vi "ROS_Wait.vi"(3 "milliseconds to wait":u32, 6 "error in":errorcluster) -> (5 "error out":errorcluster)   [LabVIEW 2010]
doc: "ROS for LV formatted wrapper for Wait(ms).vi"
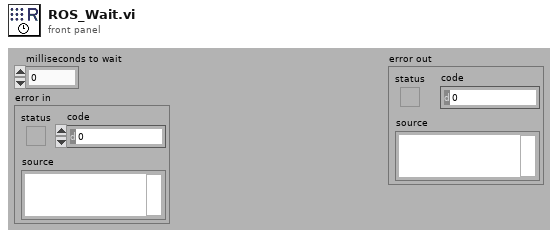
[diagram p1: front panel]
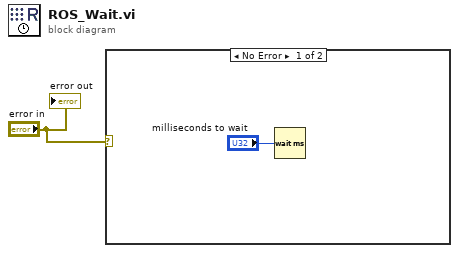
[diagram p0: block diagram]
diagram:
  n1 = case shown="No Error" "error in" {
    frame No Error {
      n2 = Wait (ms)(milliseconds to wait="milliseconds to wait") -> ()  [unwired: 1 out]
    }
    frame Error {
    }
  }
  "error out" <- "error in"
